vi "Laser Intensity Control.vi"(4 "Close?":bool, 5 "Enum":T1(ring), 7 "Intensity Control, 0~-7000 (mV)":dbl=-1000.0 format="%_8g") -> (1 "Laser Lock?":bool)   [LabVIEW 2014]
uses:
  <vilib>/Analysis/baseanly.llb/Mean (DBL).vi
  <vilib>/DAQmx/create/channels.llb/DAQmx Create Channel (AO-Voltage-Basic).vi
  <vilib>/DAQmx/write.llb/DAQmx Write (Analog 1D DBL NChan 1Samp).vi
  Main-Stage-Based/(Global) Current handle and LaserPower_YCC.vi
  <vilib>/Analysis/NI_AALBase.lvlib
panel:
  in  "Read?":bool
  in  "Centering power (mV)":dbl=-800.0
  out "Current Power (mV)":dbl format="%0.5f"
  out "Output Resolution (mV)":dbl
  # "DAC : 16 bit"
  # "-1200 mV 26.8mW"
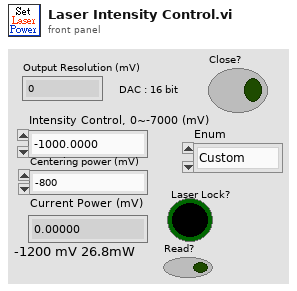
[diagram p1: front panel]
types:
  T1 = enum16{"Custom", "Centering", "1000 mV", "4500 mV"}
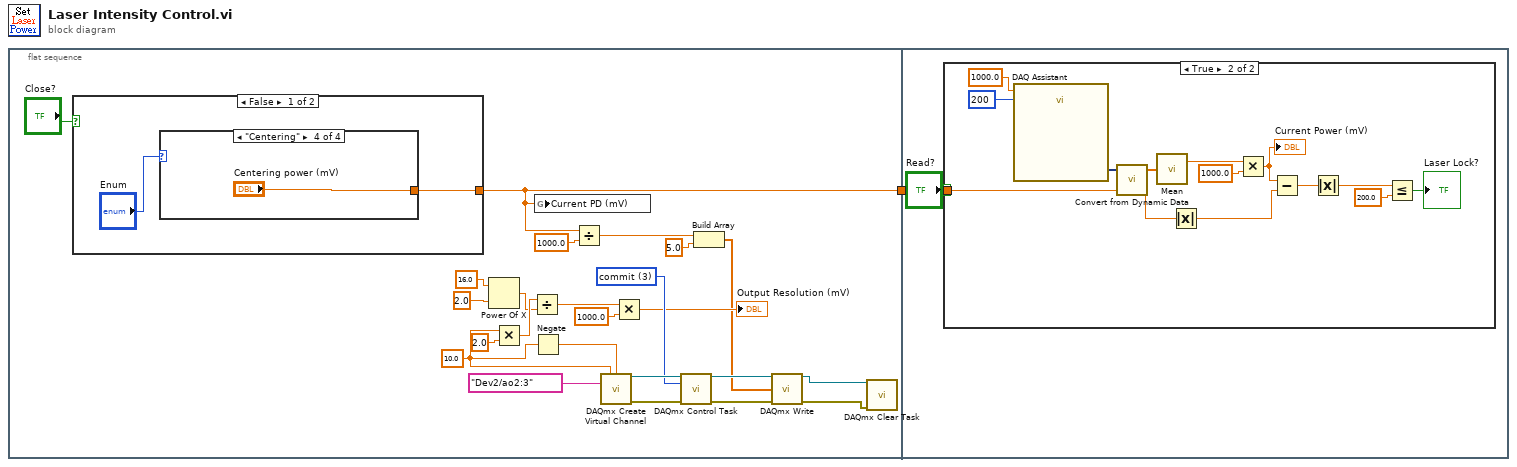
[diagram p0: block diagram]
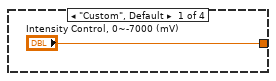
[diagram p2: hidden frame]
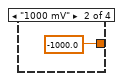
[diagram p3: hidden frame]
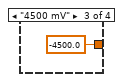
[diagram p4: hidden frame]
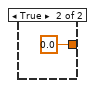
[diagram p5: hidden frame]
diagram:
  n1 = flat-sequence {
    tunnel: [w4] -> w1
    tunnel: w1 -> [w34]
    frame #0 {
      w18 = 10.0 ("maximum value")
      w22 = 3 items=["verify"=2, "reserve"=4, "commit"=3, "unreserve"=5, "abort"=6] ("action")
      n2 = case shown="False" "Close?" {
        tunnel: [w27 0.0 ("element")] -> w4
        frame False {
          n3 = case shown="\"Centering\"" "Enum" {
            tunnel: ["Intensity Control, 0~-7000 (mV)" -1000.0 ("Intensity Control, 0~-7000 (mV)") -4500.0 ("Intensity Control, 0~-7000 (mV)") "Centering power (mV)"] -> w27
            frame "Custom", Default {
            }
            frame "1000 mV" {
            }
            frame "4500 mV" {
            }
            frame "Centering" {
            }
          }
        }
        frame True {
        }
      }
      n4 = Power Of X(1:2.0 ("x"), 2:16.0 ("y")) -> (0:w13:dbl)
      n5 = Multiply(x=w18, y=2.0 ("maximum value")) -> (x*y=w16:dbl)
      n6 = Divide(x=w16, y=w13) -> (x/y=w12:dbl)
      n7 = Negate(x=w18) -> (-x=w19:dbl)
      n8 = global write "(Global) Current handle and LaserPower_YCC.vi" "Current PD (mV)"(w4) -> ()
      n9 = Divide(x=w4, y=1000.0) -> (x/y=w8:dbl)
      n10 = call-poly <vilib>:"DAQmx Create Virtual Channel.vi"("maximum value"=w18, "minimum value"=w19, "physical channels"=tag "Dev2/ao2:3") -> ("task out"=w23:refnum<k21>, "error out"=w24:errorcluster)  [unwired: 11 in]
      n11 = Multiply(x=w12, y=1000.0) -> (x*y=→"Output Resolution (mV)":dbl)
      n12 = call <vilib>:"DAQmx Control Task.vi"("task/channels in"=w23, "action"=w22, "error in"=w24) -> ("task out"=w21:refnum<k21>, "error out"=w20:errorcluster)  [unwired: 11 in]
      n13 = Build Array(w8, 5.0 ("element")) -> (w6:dbl[])
      n14 = call-poly <vilib>:"DAQmx Write.vi"("task/channels in"=w21, "data"=w6, "error in"=w20) -> ("task out"=w3:refnum<k21>, "error out"=w2:errorcluster)  [unwired: 10 in, 1 out]
      n15 = call <vilib>:"DAQmx Clear Task.vi"("task in"=w3, "error in"=w2) -> ()  [unwired: 13 in, 1 out]
    }
    frame #1 {
      n16 = case shown="True" "Read?" {
        tunnel: w34 -> [_ w36]
        frame False {
        }
        frame True {
          n17 = call "DAQ Assistant"("rate"=1000.0, "number of samples"=200) -> ("data"=w44:dynamicdata)  [unwired: 15 in, 2 out]
          n18 = call "Convert from Dynamic Data"("Dynamic Data Type"=w44) -> ("Array"=w45:dbl[])  [unwired: 3 in]
          n19 = call-poly <vilib>:"Mean.vi"("X"=w45) -> ("mean"=w47:dbl)  [unwired: 1 out]
          n20 = Absolute Value(x=w36) -> (abs(x)=w35:dbl)
          n21 = Multiply(x=w47, y=1000.0) -> (x*y=w41:dbl)
          "Current Power (mV)" <- w41
          n22 = Subtract(x=w41, y=w35) -> (x-y=w40:dbl)
          n23 = Absolute Value(x=w40) -> (abs(x)=w39:dbl)
          n24 = Less Or Equal?(x=w39, y=200.0) -> (x <= y?=→"Laser Lock?":bool)
        }
      }
    }
  }
